vi "Select Tool.vi"(7 "DUT1?":bool=TRUE, 8 "error in":errorcluster, 9 "Supply PCB over Programator":bool, 10 "Family":string, 11 "6.25":bool=TRUE) -> (0 "error out":errorcluster, 1 "Firmware passed":bool, 2 "standard error":string, 3 "standard output":string)   [LabVIEW 2023]
panel:
  out "return code":i32
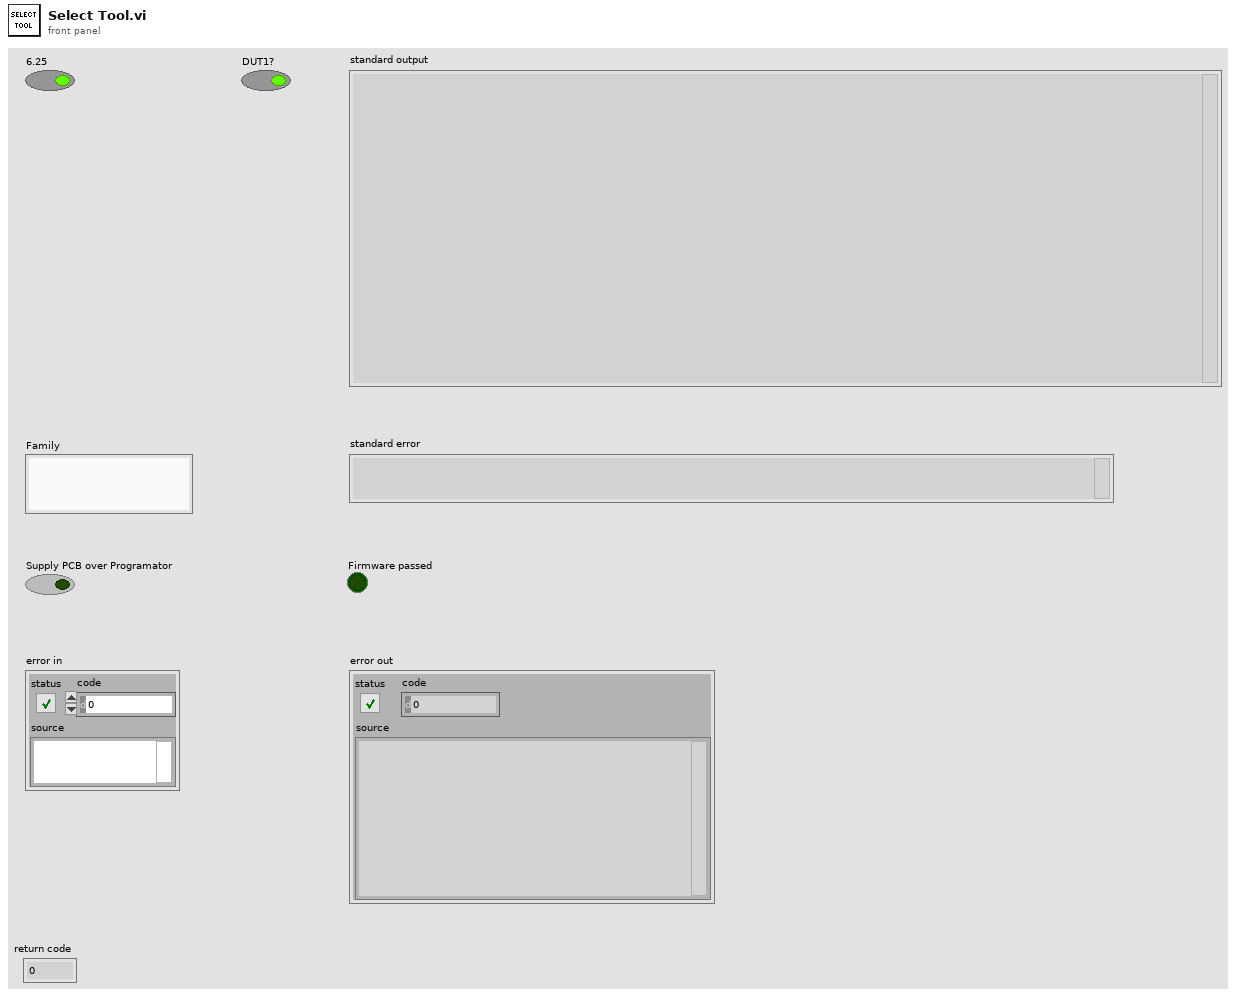
[diagram p1: front panel]
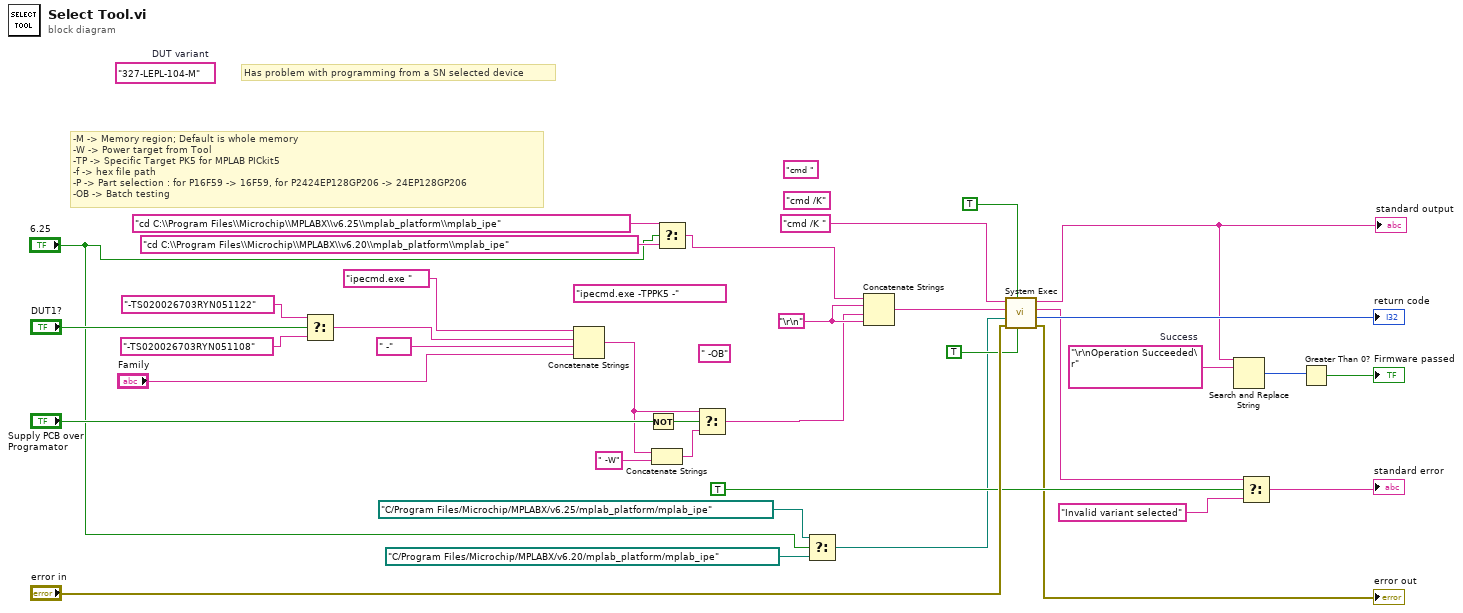
[diagram p0: block diagram]
diagram:
  (unwired) "cmd " ("command line")
  (unwired) "ipecmd.exe -TPPK5 -" ("command line")
  (unwired) "cmd /K" ("command line")
  (unwired) " -OB" ("string")
  w24 = "\r\nOperation Succeeded\r"  # Success
  (unwired) "327-LEPL-104-M"  # DUT variant
  w20 = "\r\n"
  # "Has problem with programming from a SN selected device"
  # "-M -> Memory region; Default is whole memory\n-W -> Power target from Tool\n-TP -> Specific Target PK5 for MPLAB PICkit5\n-f -> hex file path\n-P -> Part selection : for P16F59 -> 16F59, for P2424EP128GP206 -> 24EP128GP206\n-OB -> Batch testing"
  n1 = Select(t="-TS020026703RYN051122" ("command line"), s="DUT1?", f="-TS020026703RYN051108" ("command line")) -> (s? t:f=w10:string)
  n2 = Concatenate Strings("ipecmd.exe " ("command line"), w10, " -" ("command line"), "Family") -> (w16:string)
  n3 = Not(x="Supply PCB over Programator") -> (.not. x?=w31:bool)
  n4 = Concatenate Strings(w16, " -W" ("string")) -> (w18:string)
  n5 = Select(t="cd C:\\Program Files\\Microchip\\MPLABX\\v6.25\\mplab_platform\\mplab_ipe" ("command line"), s="6.25", f="cd C:\\Program Files\\Microchip\\MPLABX\\v6.20\\mplab_platform\\mplab_ipe" ("command line")) -> (s? t:f=w5:string)
  n6 = Select(t=w16, s=w31, f=w18) -> (s? t:f=w8:string)
  n7 = Select(t=path "C:/Program Files/Microchip/MPLABX/v6.25/mplab_platform/mplab_ipe" ("working directory"), s="6.25", f=path "C:/Program Files/Microchip/MPLABX/v6.20/mplab_platform/mplab_ipe" ("working directory")) -> (s? t:f=w1:path)
  n8 = Concatenate Strings(w5, w20, w8, w20) -> (w34:string)
  n9 = call <vilib>:"System Exec.vi"("run minimized? (F)"=TRUE, "wait until completion? (T)"=TRUE, "error in (no error)"="error in", "working directory"=w1, "standard input"=w34, "command line"="cmd /K ") -> ("error out"=→"error out":errorcluster, "return code"=→"return code":i32, "standard error"=w27:string, "standard output"=w25:string)  [unwired: 2 in]
  "standard output" <- w25
  n10 = Search and Replace String(input string=w25, search string=w24) -> (number of replacements=w23:i32)  [unwired: 6 in, 3 out]
  n11 = Select(t=w27, s=TRUE, f="Invalid variant selected") -> (s? t:f=→"standard error":string)
  n12 = Greater Than 0?(x=w23) -> (x > 0?=→"Firmware passed":bool)
